vi "Stop.vi"(8 "error in (no error)":errorcluster, 11 "KUKA youBot platform in":refnum<class "NI_Robotics_KUKA youBot Platform.lvclass">) -> (0 "error out":errorcluster, 3 "KUKA youBot platform out":refnum<class "NI_Robotics_KUKA youBot Platform.lvclass">)   [LabVIEW 2017, in "NI_Robotics_KUKA youBot Host.lvlib" / "NI_Robotics_KUKA youBot Platform.lvclass"]
uses:
  <vilib>/robotics/KUKA youBot/Basic Device/Mobile Platform/NI_Robotics_KUKA youBot Platform.lvclass
  <vilib>/robotics/KUKA youBot/Basic Device/Mobile Platform/NI_Robotics_KUKA youBot Platform.lvclass/NI_Robotics_KUKA youBot Platform.ctl
  <vilib>/robotics/KUKA youBot/Motor/Wheel Motor/NI_Robotics_KUKA youBot Wheel Motor.lvclass
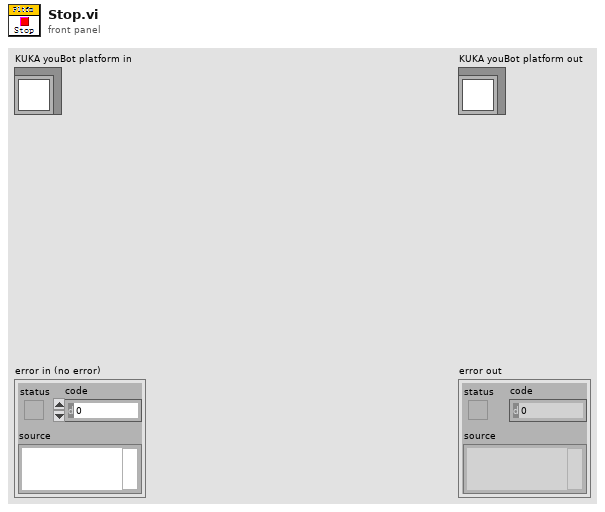
[diagram p1: front panel]
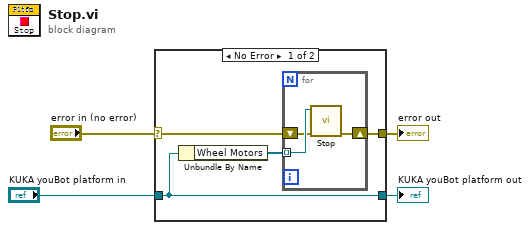
[diagram p0: block diagram]
diagram:
  n1 = case shown="No Error" "error in (no error)" {
    selector: "error in (no error)" -> [w6 w13]
    tunnel: [w5 w13] -> w3
    tunnel: [w8 w12] -> w1
    tunnel: "KUKA youBot platform in" -> [w8 w12]
    frame No Error {
      n2 = Unbundle By Name(w8) -> ("Wheel Motors"=w7:refnum<class "NI_Robotics_KUKA youBot Wheel Motor.lvclass">[])
      n3 = for {
        tunnel: w7 -> [w11] mode=indexing
        shift-right: [w9] -> w5
        shift-left: w6 -> [w10]
        n4 = call-dynamic "Stop.vi"("error in (no error)"=w10, "KUKA youBot Wheel Motor in"=w11) -> ("error out"=w9:errorcluster)  [unwired: 8 in, 1 out]
      }
    }
    frame Error {
    }
  }
  "error out" <- w3
  "KUKA youBot platform out" <- w1
